vi "ParseInputs.vi"(8 "error in (no error)":errorcluster, 10 "Inputs":string[](array[string]), 11 "DiscoverTestCases in":refnum<class "DiscoverTestCases.lvclass">) -> (0 "error out":errorcluster, 3 "DiscoverTestCases out":refnum<class "DiscoverTestCases.lvclass">)   [LabVIEW 2027, in "DiscoverTestCases.lvclass"]
uses:
  DiscoverTestCases.lvclass
  DiscoverTestCases.lvclass/DiscoverTestCases.ctl
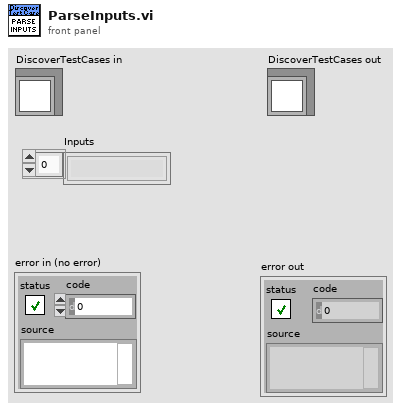
[diagram p1: front panel]
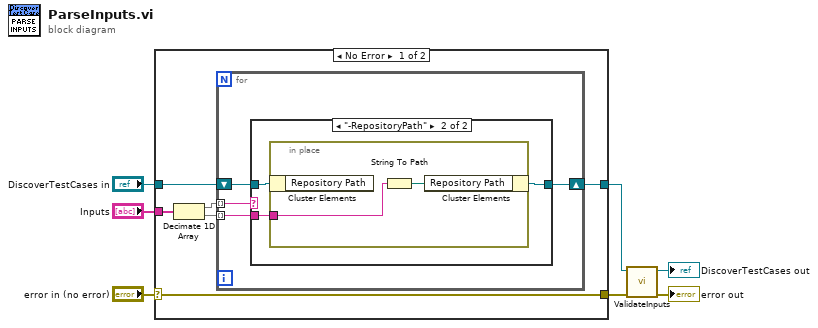
[diagram p0: block diagram]
diagram:
  n1 = case shown="No Error" "error in (no error)" {
    selector: "error in (no error)" -> [w8 w25]
    tunnel: [w8 w25] -> w2
    tunnel: "Inputs" -> [w13 _]
    tunnel: "DiscoverTestCases in" -> [w10 w24]
    tunnel: [w9 w24] -> w4
    frame No Error {
      n2 = Decimate 1D Array(w13) -> (w12:string[], w11:string[])
      n3 = for {
        tunnel: w12 -> [w17] mode=indexing
        tunnel: w11 -> [w14] mode=indexing
        shift-right: [w15] -> w9
        shift-left: w10 -> [w16]
        n4 = case shown="\"-RepositoryPath\"" w17 {
          tunnel: w16 -> [w18 w21]
          tunnel: [w18 w20] -> w15
          tunnel: w14 -> [_ w19]
          frame Default {
          }
          frame "-RepositoryPath" {
            n5 = in-place {
              in-place-border: w19 -> [w22]
              n6 = in-place-cluster #1(w21) -> ()  [unwired: 1 out]
              n7 = String To Path(string=w22) -> (path=w23:path)
              n8 = in-place-cluster #1("Repository Path"=w23) -> (w20:refnum<class "DiscoverTestCases.lvclass">)
            }
          }
        }
      }
    }
    frame Error {
    }
  }
  n9 = call "ValidateInputs.vi"("error in (no error)"=w2, "DiscoverTestCases in"=w4) -> ("error out"=→"error out":errorcluster, "DiscoverTestCases out"=→"DiscoverTestCases out":refnum<class "DiscoverTestCases.lvclass">)  [unwired: 8 in]
